vi "TSCAN_DBC_R&S.vi"(10 "Data":T4={"Communication message"={"Sender"="", "receiver"="", "message"="", "data"=variant}, "Data"={"Config_parameter"={"Bus_Type"=0, "Channel"=1, "Channels used"=1, "DLL_PATH"=path "", "Read message type"=1, "REC_Channel"=0}, "Send_parameter"={"SendData"=[0, 0, 0, 0, 0, 0, 0, 0, 0, 0, 0, 0, 0, 0, 0, 0, 0, 0, 0, 0, 0, 0, 0, 0, 0, 0, 0, 0, 0, 0, 0, 0, 0, 0, 0, 0, 0, 0, 0, 0, 0, 0, 0, 0, 0, 0, 0, 0, 0, 0, 0, 0, 0, 0, 0, 0, 0, 0, 0, 0, 0, 0, 0, 0, 0, 0, 0, 0, 0, 0, 0, 0, 0, 0, 0], "Data Length"=15, "ID"=0, "Frame Format"=0, "Frame Type"=0, "BRS"=enum."Close", "FD Frame"=0, "async&sync"=enum."async", "Timeout"=0}, "DBC_Ctr"={"DBC Path"=path "", "DBC loading channel"=0, "DatabaseId"=0, "DBMessages"=[], "DBSignals"=[]}, "CAN_Config_Array"=[], "CANFD_Config_Array"=[], "CAN_Config_Regs_Array"=[], "CANFD_Config_Regs_Array"=[], "Blf_Log"={"Blf_Log_PATH"=path ""}, "UDS"={"UDS Control"={"UDS Channel Index"=0, "Request ID"=1992, "Response ID"=2015, "Request ID (Func)"=1, "Session Mode"=1, "Reset Mode"=255, "DTC Mask"=0, "GropOfDTC"=0, "Seed Level"=2, "Seed"=[], "Key Level"=0, "Key"=[], "Read Identifier"=0, "UDS Read Data"=[], "ASCII Data"="", "Write Identifier"=0, "UDS Wrtie Data"=[], "IO Control Identifier"=1, "UDS IOControl Data"=[], "IO Control Mode"=0, "UDS IOControl Read Data"=[], "Routine Control Identifier"=0, "UDS RoutineControl Data"=[], "UDS RoutineControl Read Data"=[], "Routine Control Mode"=1, "SupportFDCAN"=TRUE, "time config"={"p2_timeout"=0, "p2_extended"=0, "s3_servertime"=0, "s3_clienttime"=0}, "ServiceLayer"={"FilledByte"=0, "STMin"=10, "BlockSize"=10, "FCDelay"=10, "MaxLength"=4095}, "Request"=[], "Respond"=[]}, "DiagModuleIndex"=1984}}, "CAN_Buffer"=[], "CANFD_Buffer"=[], "error in"={"status"=FALSE, "code"=0, "source"=""}, "CAN_Period_Datas"=[], "CANFD_period_Datas"=[], "CAN_Filtering_Datas"=[], "CANFD_Filtering_Datas"=[], "AsynCall?"=FALSE} {"Data"."UDS"."UDS Control"."Respond" format="%.0x"; "Data"."UDS"."UDS Control"."Request" format="%.0x"; "Data"."UDS"."UDS Control"."ServiceLayer"."FilledByte" format="%.0x"; "Data"."UDS"."UDS Control"."GropOfDTC" format="%.0x"; "Data"."UDS"."UDS Control"."DTC Mask" format="%.0x"; "Data"."UDS"."UDS Control"."UDS RoutineControl Read Data" format="%.0x"; "Data"."UDS"."UDS Control"."UDS RoutineControl Data" format="%.0x"; "Data"."UDS"."UDS Control"."Routine Control Identifier" format="%.0x"; "Data"."UDS"."UDS Control"."UDS IOControl Read Data" format="%.0x"; "Data"."UDS"."UDS Control"."UDS IOControl Data" format="%.0x"; "Data"."UDS"."UDS Control"."IO Control Identifier" format="%.0x"; "Data"."UDS"."UDS Control"."UDS Wrtie Data" format="%.0x"; "Data"."UDS"."UDS Control"."UDS Read Data" format="%.0x"; "Data"."UDS"."UDS Control"."Write Identifier" format="%.0x"; "Data"."UDS"."UDS Control"."Read Identifier" format="%.0x"; "Data"."UDS"."UDS Control"."Key" format="%.0x"; "Data"."UDS"."UDS Control"."Seed" format="%.0x"; "Data"."UDS"."UDS Control"."Request ID (Func)" format="%.0x"; "Data"."UDS"."UDS Control"."Response ID" format="%.0x"; "Data"."UDS"."UDS Control"."Request ID" format="%.0x"; "Data"."UDS"."UDS Control"."Session Mode" items=["DefaultSession"=1, "ProgrammingSession"=2, "ExtendedDiagnosticSession"=3]; "Data"."UDS"."UDS Control"."Reset Mode" items=["HardReset"=1, "keyOffOnReset"=2, "SoftReset"=3]; "Data"."UDS"."UDS Control"."IO Control Mode" items=["ReturnControlToECU", "ResetToDefault", "FreezeCurrentState", "ShortTermAdjustment"]; "Data"."UDS"."UDS Control"."Routine Control Mode" items=["Start routine"=1, "Stop routine"=2, "Request routine results"=3]; "Data"."CAN_Config_Regs_Array"."CAN configuration"."AAppChannel" items=["CHN1", "CHN2", "CHN3", "CHN4", "CHN5", "CHN6", "CHN7", "CHN8", "CHN9", "CHN10", "CHN11", "CHN12", "CHN13", "CHN14", "CHN15", "CHN16", "CHN17", "CHN18", "CHN19", "CHN20", "CHN21", "CHN22", "CHN23", "CHN24", "CHN25", "CHN26", "CHN27", "CHN28", "CHN29", "CHN30", "CHN31", "CHN32"]; "Data"."CAN_Config_Regs_Array"."CAN configuration"."AHwChannel" items=["CHN1", "CHN2", "CHN3", "CHN4", "CHN5", "CHN6", "CHN7", "CHN8", "CHN9", "CHN10", "CHN11", "CHN12", "CHN13", "CHN14", "CHN15", "CHN16", "CHN17", "CHN18", "CHN19", "CHN20", "CHN21", "CHN22", "CHN23", "CHN24", "CHN25", "CHN26", "CHN27", "CHN28", "CHN29", "CHN30", "CHN31", "CHN32"]; "Data"."CAN_Config_Regs_Array"."CAN configuration"."HardwareType" items=["BUS_UNKNOWN_TYPE", "TS_TCP_DEVICE", "XL_USB_DEVICE", "TS_USB_DEVICE", "PEAK_USB_DEVICE", "KVASER_USB_DEVICE", "ZLG_USB_DEVICE", "ICS_USB_DEVICE", "TS_TC1005_DEVICE", "CANABLE_USB_DEVICE", "TS_WIRELESS_OBD", "TS_USB_DEVICE_EX", "IXXAT_USB_DEVICE", "TS_ETH_IF_DEVICE", "TS_USB_IF_DEVICE", "BUS_DEV_TYPE_COUNT"]; "Data"."CANFD_Config_Regs_Array"."CANFD Configuration"."Hardware Type" items=["BUS_UNKNOWN_TYPE", "TS_TCP_DEVICE", "XL_USB_DEVICE", "TS_USB_DEVICE", "PEAK_USB_DEVICE", "KVASER_USB_DEVICE", "ZLG_USB_DEVICE", "ICS_USB_DEVICE", "TS_TC1005_DEVICE", "CANABLE_USB_DEVICE", "TS_WIRELESS_OBD", "TS_USB_DEVICE_EX", "IXXAT_USB_DEVICE", "TS_ETH_IF_DEVICE", "TS_USB_IF_DEVICE", "BUS_DEV_TYPE_COUNT"]; "Data"."CANFD_Config_Regs_Array"."CANFD Configuration"."AHwChannel" items=["CHN1", "CHN2", "CHN3", "CHN4", "CHN5", "CHN6", "CHN7", "CHN8", "CHN9", "CHN10", "CHN11", "CHN12", "CHN13", "CHN14", "CHN15", "CHN16", "CHN17", "CHN18", "CHN19", "CHN20", "CHN21", "CHN22", "CHN23", "CHN24", "CHN25", "CHN26", "CHN27", "CHN28", "CHN29", "CHN30", "CHN31", "CHN32"]; "Data"."CANFD_Config_Regs_Array"."CANFD Configuration"."AAppChannel" items=["CHN1", "CHN2", "CHN3", "CHN4", "CHN5", "CHN6", "CHN7", "CHN8", "CHN9", "CHN10", "CHN11", "CHN12", "CHN13", "CHN14", "CHN15", "CHN16", "CHN17", "CHN18", "CHN19", "CHN20", "CHN21", "CHN22", "CHN23", "CHN24", "CHN25", "CHN26", "CHN27", "CHN28", "CHN29", "CHN30", "CHN31", "CHN32"]; "Data"."CANFD_Config_Regs_Array"."CANFD Configuration"."AControllerType" items=["lfdtCAN", "lfdtISOFDCAN", "lfdtNonISOFDFDCAN"]; "Data"."CANFD_Config_Regs_Array"."CANFD Configuration"."AControllerMode" items=["lfdmNormal", "lfdmACKOff", "lfdmRestricted"]; "Data"."CANFD_Config_Array"."Hardware Type" items=["BUS_UNKNOWN_TYPE", "TS_TCP_DEVICE", "XL_USB_DEVICE", "TS_USB_DEVICE", "PEAK_USB_DEVICE", "KVASER_USB_DEVICE", "ZLG_USB_DEVICE", "ICS_USB_DEVICE", "TS_TC1005_DEVICE", "CANABLE_USB_DEVICE", "TS_WIRELESS_OBD", "TS_USB_DEVICE_EX", "IXXAT_USB_DEVICE", "TS_ETH_IF_DEVICE", "TS_USB_IF_DEVICE", "BUS_DEV_TYPE_COUNT"]; "Data"."CANFD_Config_Array"."AHwChannel" items=["CHN1", "CHN2", "CHN3", "CHN4", "CHN5", "CHN6", "CHN7", "CHN8", "CHN9", "CHN10", "CHN11", "CHN12", "CHN13", "CHN14", "CHN15", "CHN16", "CHN17", "CHN18", "CHN19", "CHN20", "CHN21", "CHN22", "CHN23", "CHN24", "CHN25", "CHN26", "CHN27", "CHN28", "CHN29", "CHN30", "CHN31", "CHN32"]; "Data"."CANFD_Config_Array"."AAppChannel" items=["CHN1", "CHN2", "CHN3", "CHN4", "CHN5", "CHN6", "CHN7", "CHN8", "CHN9", "CHN10", "CHN11", "CHN12", "CHN13", "CHN14", "CHN15", "CHN16", "CHN17", "CHN18", "CHN19", "CHN20", "CHN21", "CHN22", "CHN23", "CHN24", "CHN25", "CHN26", "CHN27", "CHN28", "CHN29", "CHN30", "CHN31", "CHN32"]; "Data"."CANFD_Config_Array"."AControllerType" items=["lfdtCAN", "lfdtISOFDCAN", "lfdtNonISOFDFDCAN"]; "Data"."CANFD_Config_Array"."AControllerMode" items=["lfdmNormal", "lfdmACKOff", "lfdmRestricted"]; "Data"."CAN_Config_Array"."AAppChannel" items=["CHN1", "CHN2", "CHN3", "CHN4", "CHN5", "CHN6", "CHN7", "CHN8", "CHN9", "CHN10", "CHN11", "CHN12", "CHN13", "CHN14", "CHN15", "CHN16", "CHN17", "CHN18", "CHN19", "CHN20", "CHN21", "CHN22", "CHN23", "CHN24", "CHN25", "CHN26", "CHN27", "CHN28", "CHN29", "CHN30", "CHN31", "CHN32"]; "Data"."CAN_Config_Array"."AHwChannel" items=["CHN1", "CHN2", "CHN3", "CHN4", "CHN5", "CHN6", "CHN7", "CHN8", "CHN9", "CHN10", "CHN11", "CHN12", "CHN13", "CHN14", "CHN15", "CHN16", "CHN17", "CHN18", "CHN19", "CHN20", "CHN21", "CHN22", "CHN23", "CHN24", "CHN25", "CHN26", "CHN27", "CHN28", "CHN29", "CHN30", "CHN31", "CHN32"]; "Data"."CAN_Config_Array"."HardwareType" items=["BUS_UNKNOWN_TYPE", "TS_TCP_DEVICE", "XL_USB_DEVICE", "TS_USB_DEVICE", "PEAK_USB_DEVICE", "KVASER_USB_DEVICE", "ZLG_USB_DEVICE", "ICS_USB_DEVICE", "TS_TC1005_DEVICE", "CANABLE_USB_DEVICE", "TS_WIRELESS_OBD", "TS_USB_DEVICE_EX", "IXXAT_USB_DEVICE", "TS_ETH_IF_DEVICE", "TS_USB_IF_DEVICE", "BUS_DEV_TYPE_COUNT"]; "Data"."DBC_Ctr"."DBSignals"."SignalList"."Message_Type" items=["CAN", "CANFD", "J1939"]; "Data"."DBC_Ctr"."DBSignals"."SignalList"."Mux_Type" items=["Normal", "multiplexor", "multiplexed"]; "Data"."DBC_Ctr"."DBSignals"."SignalList"."Is_Motorola" items=["Intel", "Motorola"]; "Data"."DBC_Ctr"."DBSignals"."SignalList"."Value_Type" items=["unsigned int", "signed int", "float", "double"]; "Data"."DBC_Ctr"."DBSignals"."SignalList"."ID" format="%.0x"; "Data"."DBC_Ctr"."DBMessages"."BRS" items=["No BRS", "BRS"]; "Data"."DBC_Ctr"."DBMessages"."ID" format="%.0x"; "Data"."DBC_Ctr"."DBMessages"."Type" items=["cftStdCAN", "cftExtCAN", "cftJ1939", "cftStdCANFD", "cftExtCANFD"]; "Data"."DBC_Ctr"."DBC loading channel" items=["CHN1", "CHN2", "CHN3", "CHN4", "CHN5", "CHN6", "CHN7", "CHN8", "CHN9", "CHN10", "CHN11", "CHN12", "CHN13", "CHN14", "CHN15", "CHN16", "CHN17", "CHN18", "CHN19", "CHN20", "CHN21", "CHN22", "CHN23", "CHN24", "CHN25", "CHN26", "CHN27", "CHN28", "CHN29", "CHN30", "CHN31", "CHN32"]; "Data"."Send_parameter"."FD Frame" items=["Ordinary CAN Data", "FD CAN Data"]; "Data"."Send_parameter"."Frame Type" items=["Standard Frame", "Extended Frame"]; "Data"."Send_parameter"."Frame Format" items=["Standard Frame", "Extended Frame"]; "Data"."Send_parameter"."ID" format="%x"; "Data"."Send_parameter"."Data Length" items=["0", "1", "2", "3", "4", "5", "6", "7", "8", "12", "16", "20", "24", "32", "48", "64"]; "Data"."Send_parameter"."SendData" format="%x"; "Data"."Config_parameter"."REC_Channel" items=["CHN1", "CHN2", "CHN3", "CHN4", "CHN5", "CHN6", "CHN7", "CHN8", "CHN9", "CHN10", "CHN11", "CHN12", "CHN13", "CHN14", "CHN15", "CHN16", "CHN17", "CHN18", "CHN19", "CHN20", "CHN21", "CHN22", "CHN23", "CHN24", "CHN25", "CHN26", "CHN27", "CHN28", "CHN29", "CHN30", "CHN31", "CHN32"]; "Data"."Config_parameter"."Read message type" items=["Only read received messages", "Receive&send messages"]; "Data"."Config_parameter"."Channels used" items=["1 Channel"=1, "2 Channels"=2, "3 Channels"=3, "4 Channels"=4, "5 Channels"=5, "6 Channels"=6, "7 Channels"=7, "8 Channels"=8, "9 Channels"=9, "10 Channels"=10, "11 Channels"=11, "12 Channels"=12, "13 Channels"=13, "14 Channels"=14, "15 Channels"=15, "16 Channels"=16]; "Data"."Config_parameter"."Channel" items=["Disable", "Enable"]; "Data"."Config_parameter"."Bus_Type" items=["CAN", "CANFD"]}, 11 "Sender":string="Demo") -> (2 "Data 2":T4={"Communication message"={"Sender"="", "receiver"="", "message"="", "data"=variant}, "Data"={"Config_parameter"={"Bus_Type"=0, "Channel"=1, "Channels used"=1, "DLL_PATH"=path "", "Read message type"=1, "REC_Channel"=0}, "Send_parameter"={"SendData"=[0, 0, 0, 0, 0, 0, 0, 0, 0, 0, 0, 0, 0, 0, 0, 0, 0, 0, 0, 0, 0, 0, 0, 0, 0, 0, 0, 0, 0, 0, 0, 0, 0, 0, 0, 0, 0, 0, 0, 0, 0, 0, 0, 0, 0, 0, 0, 0, 0, 0, 0, 0, 0, 0, 0, 0, 0, 0, 0, 0, 0, 0, 0, 0, 0, 0, 0, 0, 0, 0, 0, 0, 0, 0, 0], "Data Length"=15, "ID"=0, "Frame Format"=0, "Frame Type"=0, "BRS"=enum."Close", "FD Frame"=0, "async&sync"=enum."async", "Timeout"=0}, "DBC_Ctr"={"DBC Path"=path "", "DBC loading channel"=0, "DatabaseId"=0, "DBMessages"=[], "DBSignals"=[]}, "CAN_Config_Array"=[], "CANFD_Config_Array"=[], "CAN_Config_Regs_Array"=[], "CANFD_Config_Regs_Array"=[], "Blf_Log"={"Blf_Log_PATH"=path ""}, "UDS"={"UDS Control"={"UDS Channel Index"=0, "Request ID"=1992, "Response ID"=2015, "Request ID (Func)"=1, "Session Mode"=1, "Reset Mode"=255, "DTC Mask"=0, "GropOfDTC"=0, "Seed Level"=2, "Seed"=[], "Key Level"=0, "Key"=[], "Read Identifier"=0, "UDS Read Data"=[], "ASCII Data"="", "Write Identifier"=0, "UDS Wrtie Data"=[], "IO Control Identifier"=1, "UDS IOControl Data"=[], "IO Control Mode"=0, "UDS IOControl Read Data"=[], "Routine Control Identifier"=0, "UDS RoutineControl Data"=[], "UDS RoutineControl Read Data"=[], "Routine Control Mode"=1, "SupportFDCAN"=TRUE, "time config"={"p2_timeout"=0, "p2_extended"=0, "s3_servertime"=0, "s3_clienttime"=0}, "ServiceLayer"={"FilledByte"=0, "STMin"=10, "BlockSize"=10, "FCDelay"=10, "MaxLength"=4095}, "Request"=[], "Respond"=[]}, "DiagModuleIndex"=1984}}, "CAN_Buffer"=[], "CANFD_Buffer"=[], "error in"={"status"=FALSE, "code"=0, "source"=""}, "CAN_Period_Datas"=[], "CANFD_period_Datas"=[], "CAN_Filtering_Datas"=[], "CANFD_Filtering_Datas"=[], "AsynCall?"=FALSE} {"Data"."UDS"."UDS Control"."Respond" format="%.0x"; "Data"."UDS"."UDS Control"."Request" format="%.0x"; "Data"."UDS"."UDS Control"."ServiceLayer"."FilledByte" format="%.0x"; "Data"."UDS"."UDS Control"."GropOfDTC" format="%.0x"; "Data"."UDS"."UDS Control"."DTC Mask" format="%.0x"; "Data"."UDS"."UDS Control"."UDS RoutineControl Read Data" format="%.0x"; "Data"."UDS"."UDS Control"."UDS RoutineControl Data" format="%.0x"; "Data"."UDS"."UDS Control"."Routine Control Identifier" format="%.0x"; "Data"."UDS"."UDS Control"."UDS IOControl Read Data" format="%.0x"; "Data"."UDS"."UDS Control"."UDS IOControl Data" format="%.0x"; "Data"."UDS"."UDS Control"."IO Control Identifier" format="%.0x"; "Data"."UDS"."UDS Control"."UDS Wrtie Data" format="%.0x"; "Data"."UDS"."UDS Control"."UDS Read Data" format="%.0x"; "Data"."UDS"."UDS Control"."Write Identifier" format="%.0x"; "Data"."UDS"."UDS Control"."Read Identifier" format="%.0x"; "Data"."UDS"."UDS Control"."Key" format="%.0x"; "Data"."UDS"."UDS Control"."Seed" format="%.0x"; "Data"."UDS"."UDS Control"."Request ID (Func)" format="%.0x"; "Data"."UDS"."UDS Control"."Response ID" format="%.0x"; "Data"."UDS"."UDS Control"."Request ID" format="%.0x"; "Data"."UDS"."UDS Control"."Session Mode" items=["DefaultSession"=1, "ProgrammingSession"=2, "ExtendedDiagnosticSession"=3]; "Data"."UDS"."UDS Control"."Reset Mode" items=["HardReset"=1, "keyOffOnReset"=2, "SoftReset"=3]; "Data"."UDS"."UDS Control"."IO Control Mode" items=["ReturnControlToECU", "ResetToDefault", "FreezeCurrentState", "ShortTermAdjustment"]; "Data"."UDS"."UDS Control"."Routine Control Mode" items=["Start routine"=1, "Stop routine"=2, "Request routine results"=3]; "Data"."CAN_Config_Regs_Array"."CAN configuration"."AAppChannel" items=["CHN1", "CHN2", "CHN3", "CHN4", "CHN5", "CHN6", "CHN7", "CHN8", "CHN9", "CHN10", "CHN11", "CHN12", "CHN13", "CHN14", "CHN15", "CHN16", "CHN17", "CHN18", "CHN19", "CHN20", "CHN21", "CHN22", "CHN23", "CHN24", "CHN25", "CHN26", "CHN27", "CHN28", "CHN29", "CHN30", "CHN31", "CHN32"]; "Data"."CAN_Config_Regs_Array"."CAN configuration"."AHwChannel" items=["CHN1", "CHN2", "CHN3", "CHN4", "CHN5", "CHN6", "CHN7", "CHN8", "CHN9", "CHN10", "CHN11", "CHN12", "CHN13", "CHN14", "CHN15", "CHN16", "CHN17", "CHN18", "CHN19", "CHN20", "CHN21", "CHN22", "CHN23", "CHN24", "CHN25", "CHN26", "CHN27", "CHN28", "CHN29", "CHN30", "CHN31", "CHN32"]; "Data"."CAN_Config_Regs_Array"."CAN configuration"."HardwareType" items=["BUS_UNKNOWN_TYPE", "TS_TCP_DEVICE", "XL_USB_DEVICE", "TS_USB_DEVICE", "PEAK_USB_DEVICE", "KVASER_USB_DEVICE", "ZLG_USB_DEVICE", "ICS_USB_DEVICE", "TS_TC1005_DEVICE", "CANABLE_USB_DEVICE", "TS_WIRELESS_OBD", "TS_USB_DEVICE_EX", "IXXAT_USB_DEVICE", "TS_ETH_IF_DEVICE", "TS_USB_IF_DEVICE", "BUS_DEV_TYPE_COUNT"]; "Data"."CANFD_Config_Regs_Array"."CANFD Configuration"."Hardware Type" items=["BUS_UNKNOWN_TYPE", "TS_TCP_DEVICE", "XL_USB_DEVICE", "TS_USB_DEVICE", "PEAK_USB_DEVICE", "KVASER_USB_DEVICE", "ZLG_USB_DEVICE", "ICS_USB_DEVICE", "TS_TC1005_DEVICE", "CANABLE_USB_DEVICE", "TS_WIRELESS_OBD", "TS_USB_DEVICE_EX", "IXXAT_USB_DEVICE", "TS_ETH_IF_DEVICE", "TS_USB_IF_DEVICE", "BUS_DEV_TYPE_COUNT"]; "Data"."CANFD_Config_Regs_Array"."CANFD Configuration"."AHwChannel" items=["CHN1", "CHN2", "CHN3", "CHN4", "CHN5", "CHN6", "CHN7", "CHN8", "CHN9", "CHN10", "CHN11", "CHN12", "CHN13", "CHN14", "CHN15", "CHN16", "CHN17", "CHN18", "CHN19", "CHN20", "CHN21", "CHN22", "CHN23", "CHN24", "CHN25", "CHN26", "CHN27", "CHN28", "CHN29", "CHN30", "CHN31", "CHN32"]; "Data"."CANFD_Config_Regs_Array"."CANFD Configuration"."AAppChannel" items=["CHN1", "CHN2", "CHN3", "CHN4", "CHN5", "CHN6", "CHN7", "CHN8", "CHN9", "CHN10", "CHN11", "CHN12", "CHN13", "CHN14", "CHN15", "CHN16", "CHN17", "CHN18", "CHN19", "CHN20", "CHN21", "CHN22", "CHN23", "CHN24", "CHN25", "CHN26", "CHN27", "CHN28", "CHN29", "CHN30", "CHN31", "CHN32"]; "Data"."CANFD_Config_Regs_Array"."CANFD Configuration"."AControllerType" items=["lfdtCAN", "lfdtISOFDCAN", "lfdtNonISOFDFDCAN"]; "Data"."CANFD_Config_Regs_Array"."CANFD Configuration"."AControllerMode" items=["lfdmNormal", "lfdmACKOff", "lfdmRestricted"]; "Data"."CANFD_Config_Array"."Hardware Type" items=["BUS_UNKNOWN_TYPE", "TS_TCP_DEVICE", "XL_USB_DEVICE", "TS_USB_DEVICE", "PEAK_USB_DEVICE", "KVASER_USB_DEVICE", "ZLG_USB_DEVICE", "ICS_USB_DEVICE", "TS_TC1005_DEVICE", "CANABLE_USB_DEVICE", "TS_WIRELESS_OBD", "TS_USB_DEVICE_EX", "IXXAT_USB_DEVICE", "TS_ETH_IF_DEVICE", "TS_USB_IF_DEVICE", "BUS_DEV_TYPE_COUNT"]; "Data"."CANFD_Config_Array"."AHwChannel" items=["CHN1", "CHN2", "CHN3", "CHN4", "CHN5", "CHN6", "CHN7", "CHN8", "CHN9", "CHN10", "CHN11", "CHN12", "CHN13", "CHN14", "CHN15", "CHN16", "CHN17", "CHN18", "CHN19", "CHN20", "CHN21", "CHN22", "CHN23", "CHN24", "CHN25", "CHN26", "CHN27", "CHN28", "CHN29", "CHN30", "CHN31", "CHN32"]; "Data"."CANFD_Config_Array"."AAppChannel" items=["CHN1", "CHN2", "CHN3", "CHN4", "CHN5", "CHN6", "CHN7", "CHN8", "CHN9", "CHN10", "CHN11", "CHN12", "CHN13", "CHN14", "CHN15", "CHN16", "CHN17", "CHN18", "CHN19", "CHN20", "CHN21", "CHN22", "CHN23", "CHN24", "CHN25", "CHN26", "CHN27", "CHN28", "CHN29", "CHN30", "CHN31", "CHN32"]; "Data"."CANFD_Config_Array"."AControllerType" items=["lfdtCAN", "lfdtISOFDCAN", "lfdtNonISOFDFDCAN"]; "Data"."CANFD_Config_Array"."AControllerMode" items=["lfdmNormal", "lfdmACKOff", "lfdmRestricted"]; "Data"."CAN_Config_Array"."AAppChannel" items=["CHN1", "CHN2", "CHN3", "CHN4", "CHN5", "CHN6", "CHN7", "CHN8", "CHN9", "CHN10", "CHN11", "CHN12", "CHN13", "CHN14", "CHN15", "CHN16", "CHN17", "CHN18", "CHN19", "CHN20", "CHN21", "CHN22", "CHN23", "CHN24", "CHN25", "CHN26", "CHN27", "CHN28", "CHN29", "CHN30", "CHN31", "CHN32"]; "Data"."CAN_Config_Array"."AHwChannel" items=["CHN1", "CHN2", "CHN3", "CHN4", "CHN5", "CHN6", "CHN7", "CHN8", "CHN9", "CHN10", "CHN11", "CHN12", "CHN13", "CHN14", "CHN15", "CHN16", "CHN17", "CHN18", "CHN19", "CHN20", "CHN21", "CHN22", "CHN23", "CHN24", "CHN25", "CHN26", "CHN27", "CHN28", "CHN29", "CHN30", "CHN31", "CHN32"]; "Data"."CAN_Config_Array"."HardwareType" items=["BUS_UNKNOWN_TYPE", "TS_TCP_DEVICE", "XL_USB_DEVICE", "TS_USB_DEVICE", "PEAK_USB_DEVICE", "KVASER_USB_DEVICE", "ZLG_USB_DEVICE", "ICS_USB_DEVICE", "TS_TC1005_DEVICE", "CANABLE_USB_DEVICE", "TS_WIRELESS_OBD", "TS_USB_DEVICE_EX", "IXXAT_USB_DEVICE", "TS_ETH_IF_DEVICE", "TS_USB_IF_DEVICE", "BUS_DEV_TYPE_COUNT"]; "Data"."DBC_Ctr"."DBSignals"."SignalList"."Message_Type" items=["CAN", "CANFD", "J1939"]; "Data"."DBC_Ctr"."DBSignals"."SignalList"."Mux_Type" items=["Normal", "multiplexor", "multiplexed"]; "Data"."DBC_Ctr"."DBSignals"."SignalList"."Is_Motorola" items=["Intel", "Motorola"]; "Data"."DBC_Ctr"."DBSignals"."SignalList"."Value_Type" items=["unsigned int", "signed int", "float", "double"]; "Data"."DBC_Ctr"."DBSignals"."SignalList"."ID" format="%.0x"; "Data"."DBC_Ctr"."DBMessages"."BRS" items=["No BRS", "BRS"]; "Data"."DBC_Ctr"."DBMessages"."ID" format="%.0x"; "Data"."DBC_Ctr"."DBMessages"."Type" items=["cftStdCAN", "cftExtCAN", "cftJ1939", "cftStdCANFD", "cftExtCANFD"]; "Data"."DBC_Ctr"."DBC loading channel" items=["CHN1", "CHN2", "CHN3", "CHN4", "CHN5", "CHN6", "CHN7", "CHN8", "CHN9", "CHN10", "CHN11", "CHN12", "CHN13", "CHN14", "CHN15", "CHN16", "CHN17", "CHN18", "CHN19", "CHN20", "CHN21", "CHN22", "CHN23", "CHN24", "CHN25", "CHN26", "CHN27", "CHN28", "CHN29", "CHN30", "CHN31", "CHN32"]; "Data"."Send_parameter"."FD Frame" items=["Ordinary CAN Data", "FD CAN Data"]; "Data"."Send_parameter"."Frame Type" items=["Standard Frame", "Extended Frame"]; "Data"."Send_parameter"."Frame Format" items=["Standard Frame", "Extended Frame"]; "Data"."Send_parameter"."ID" format="%x"; "Data"."Send_parameter"."Data Length" items=["0", "1", "2", "3", "4", "5", "6", "7", "8", "12", "16", "20", "24", "32", "48", "64"]; "Data"."Send_parameter"."SendData" format="%x"; "Data"."Config_parameter"."REC_Channel" items=["CHN1", "CHN2", "CHN3", "CHN4", "CHN5", "CHN6", "CHN7", "CHN8", "CHN9", "CHN10", "CHN11", "CHN12", "CHN13", "CHN14", "CHN15", "CHN16", "CHN17", "CHN18", "CHN19", "CHN20", "CHN21", "CHN22", "CHN23", "CHN24", "CHN25", "CHN26", "CHN27", "CHN28", "CHN29", "CHN30", "CHN31", "CHN32"]; "Data"."Config_parameter"."Read message type" items=["Only read received messages", "Receive&send messages"]; "Data"."Config_parameter"."Channels used" items=["1 Channel"=1, "2 Channels"=2, "3 Channels"=3, "4 Channels"=4, "5 Channels"=5, "6 Channels"=6, "7 Channels"=7, "8 Channels"=8, "9 Channels"=9, "10 Channels"=10, "11 Channels"=11, "12 Channels"=12, "13 Channels"=13, "14 Channels"=14, "15 Channels"=15, "16 Channels"=16]; "Data"."Config_parameter"."Channel" items=["Disable", "Enable"]; "Data"."Config_parameter"."Bus_Type" items=["CAN", "CANFD"]})   [LabVIEW 2014]
uses:
  <vilib>/Utility/miscctls.llb/LVPointTypeDef.ctl
  Typedef/TLibCANFD.ctl
  Typedef/TLibCAN.ctl
  Typedef/TSCAN_Config_parameter.ctl
  Typedef/TSCAN_Send_parameter.ctl
  DataBase/Typedef/DBMessage.ctl
  DataBase/Typedef/DBSignal.ctl
  Typedef/TSCAN_DBC_Ctr.ctl
  All_Control/Typedef/Hardware Type.ctl
  Utilities/Typedef/Hardware_Subtype.ctl
  Typedef/TSCAN_CAN_Configuration.ctl
  Typedef/TSCAN_CANFD_Configuration.ctl
  Typedef/TSCAN_CANFD_Configuration_Regs.ctl
  Typedef/TSCAN_CAN_Configuration_Regs.ctl
  All_Control/Typedef/Blf_Log.ctl
  Diagnosis/Typedef/UDS Control.ctl
  Diagnosis/Typedef/UDS Cluster.ctl
  Typedef/TSCAN_CAN_CANFD_Demo_Data.ctl
  Typedef/TSCAN_CAN_CANFD_Demo_Data1.ctl
panel:
  out "Type":T1(ring)
  in  "Channel":i32(ring) items=["CHN1", "CHN2", "CHN3", "CHN4", "CHN5", "CHN6", "CHN7", "CHN8", "CHN9", "CHN10", "CHN11", "CHN12", "CHN13", "CHN14", "CHN15", "CHN16", "CHN17", "CHN18", "CHN19", "CHN20", "CHN21", "CHN22", "CHN23", "CHN24", "CHN25", "CHN26", "CHN27", "CHN28", "CHN29", "CHN30", "CHN31", "CHN32"]
  in  "Send":bool
  out "CANFD Data":T2 {"FIdentifier" format="%x"}
  out "CAN Data":T3 {"FIdentifier" format="%x"}
  in  "Signals":string[][](array[string])
  in  "Messages":string(combo)
  in  "Creat error":bool
  in  "log":i32(listbox)
  in  "Quit":bool
  # "Name"
  # "Value"
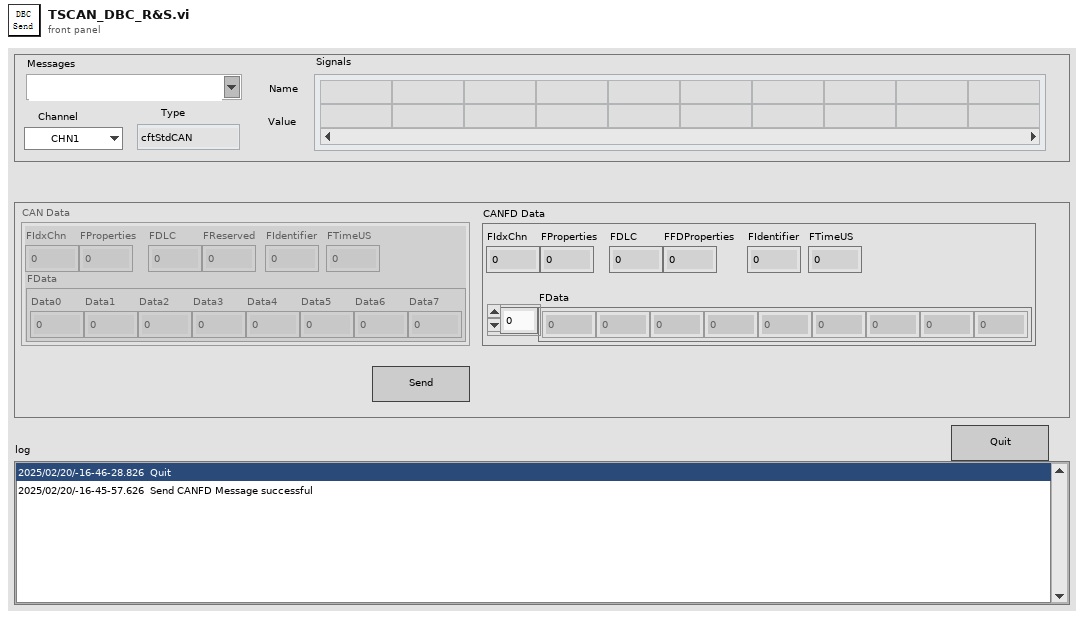
[diagram p1: front panel]
types:
  T1 = enum16{"cftStdCAN", "cftExtCAN", "cftJ1939", "cftStdCANFD", "cftExtCANFD"}
  T2 = cluster{"FIdxChn":u8, "FProperties":u8, "FDLC":u8, "FFDProperties":u8, "FIdentifier":i32, "FTimeUS":u64, "FData":dbl[]}
  T3 = cluster{"FIdxChn":u8, "FProperties":u8, "FDLC":u8, "FReserved":u8, "FIdentifier":i32, "FTimeUS":u64, "FData":cluster{"Data0":u8, "Data1":u8, "Data2":u8, "Data3":u8, "Data4":u8, "Data5":u8, "Data6":u8, "Data7":u8}}
  T4 = typedef "TSCAN_CAN_CANFD_Demo_Data1.ctl" = cluster{"Communication message":cluster{"Sender":string, "receiver":string, "message":string, "data":variant}, "Data":T5, "CAN_Buffer":cluster{"FIdxChn":u8, "FProperties":u8, "FDLC":u8, "FReserved":u8, "FIdentifier":i32, "FTimeUS":u64, "FData":cluster{"Data0":u8, "Data1":u8, "Data2":u8, "Data3":u8, "Data4":u8, "Data5":u8, "Data6":u8, "Data7":u8}}[], "CANFD_Buffer":cluster{"FIdxChn":u8, "FProperties":u8, "FDLC":u8, "FReserved":u8, "FIdentifier":i32, "FTimeUS":u64, "FDatas":cluster{"Initialize array[0]":u8, "Initialize array[1]":u8, "Initialize array[2]":u8, "Initialize array[3]":u8, "Initialize array[4]":u8, "Initialize array[5]":u8, "Initialize array[6]":u8, "Initialize array[7]":u8, "Initialize array[8]":u8, "Initialize array[9]":u8, "Initialize array[10]":u8, "Initialize array[11]":u8, "Initialize array[12]":u8, "Initialize array[13]":u8, "Initialize array[14]":u8, "Initialize array[15]":u8, "Initialize array[16]":u8, "Initialize array[17]":u8, "Initialize array[18]":u8, "Initialize array[19]":u8, "Initialize array[20]":u8, "Initialize array[21]":u8, "Initialize array[22]":u8, "Initialize array[23]":u8, "Initialize array[24]":u8, "Initialize array[25]":u8, "Initialize array[26]":u8, "Initialize array[27]":u8, "Initialize array[28]":u8, "Initialize array[29]":u8, "Initialize array[30]":u8, "Initialize array[31]":u8, "Initialize array[32]":u8, "Initialize array[33]":u8, "Initialize array[34]":u8, "Initialize array[35]":u8, "Initialize array[36]":u8, "Initialize array[37]":u8, "Initialize array[38]":u8, "Initialize array[39]":u8, "Initialize array[40]":u8, "Initialize array[41]":u8, "Initialize array[42]":u8, "Initialize array[43]":u8, "Initialize array[44]":u8, "Initialize array[45]":u8, "Initialize array[46]":u8, "Initialize array[47]":u8, "Initialize array[48]":u8, "Initialize array[49]":u8, "Initialize array[50]":u8, "Initialize array[51]":u8, "Initialize array[52]":u8, "Initialize array[53]":u8, "Initialize array[54]":u8, "Initialize array[55]":u8, "Initialize array[56]":u8, "Initialize array[57]":u8, "Initialize array[58]":u8, "Initialize array[59]":u8, "Initialize array[60]":u8, "Initialize array[61]":u8, "Initialize array[62]":u8, "Initialize array[63]":u8}}[], "error in":errorcluster, "CAN_Period_Datas":cluster{"FIdxChn":u8, "FProperties":u8, "FDLC":u8, "FReserved":u8, "FIdentifier":i32, "FTimeUS":u64, "FData":cluster{"Data0":u8, "Data1":u8, "Data2":u8, "Data3":u8, "Data4":u8, "Data5":u8, "Data6":u8, "Data7":u8}}[], "CANFD_period_Datas":cluster{"FIdxChn":u8, "FProperties":u8, "FDLC":u8, "FReserved":u8, "FIdentifier":i32, "FTimeUS":u64, "FDatas":cluster{"Initialize array[0]":u8, "Initialize array[1]":u8, "Initialize array[2]":u8, "Initialize array[3]":u8, "Initialize array[4]":u8, "Initialize array[5]":u8, "Initialize array[6]":u8, "Initialize array[7]":u8, "Initialize array[8]":u8, "Initialize array[9]":u8, "Initialize array[10]":u8, "Initialize array[11]":u8, "Initialize array[12]":u8, "Initialize array[13]":u8, "Initialize array[14]":u8, "Initialize array[15]":u8, "Initialize array[16]":u8, "Initialize array[17]":u8, "Initialize array[18]":u8, "Initialize array[19]":u8, "Initialize array[20]":u8, "Initialize array[21]":u8, "Initialize array[22]":u8, "Initialize array[23]":u8, "Initialize array[24]":u8, "Initialize array[25]":u8, "Initialize array[26]":u8, "Initialize array[27]":u8, "Initialize array[28]":u8, "Initialize array[29]":u8, "Initialize array[30]":u8, "Initialize array[31]":u8, "Initialize array[32]":u8, "Initialize array[33]":u8, "Initialize array[34]":u8, "Initialize array[35]":u8, "Initialize array[36]":u8, "Initialize array[37]":u8, "Initialize array[38]":u8, "Initialize array[39]":u8, "Initialize array[40]":u8, "Initialize array[41]":u8, "Initialize array[42]":u8, "Initialize array[43]":u8, "Initialize array[44]":u8, "Initialize array[45]":u8, "Initialize array[46]":u8, "Initialize array[47]":u8, "Initialize array[48]":u8, "Initialize array[49]":u8, "Initialize array[50]":u8, "Initialize array[51]":u8, "Initialize array[52]":u8, "Initialize array[53]":u8, "Initialize array[54]":u8, "Initialize array[55]":u8, "Initialize array[56]":u8, "Initialize array[57]":u8, "Initialize array[58]":u8, "Initialize array[59]":u8, "Initialize array[60]":u8, "Initialize array[61]":u8, "Initialize array[62]":u8, "Initialize array[63]":u8}}[], "CAN_Filtering_Datas":cluster{"FIdxChn":u8, "FProperties":u8, "FDLC":u8, "FReserved":u8, "FIdentifier":i32, "FTimeUS":u64, "FData":cluster{"Data0":u8, "Data1":u8, "Data2":u8, "Data3":u8, "Data4":u8, "Data5":u8, "Data6":u8, "Data7":u8}}[], "CANFD_Filtering_Datas":cluster{"FIdxChn":u8, "FProperties":u8, "FDLC":u8, "FReserved":u8, "FIdentifier":i32, "FTimeUS":u64, "FDatas":cluster{"Initialize array[0]":u8, "Initialize array[1]":u8, "Initialize array[2]":u8, "Initialize array[3]":u8, "Initialize array[4]":u8, "Initialize array[5]":u8, "Initialize array[6]":u8, "Initialize array[7]":u8, "Initialize array[8]":u8, "Initialize array[9]":u8, "Initialize array[10]":u8, "Initialize array[11]":u8, "Initialize array[12]":u8, "Initialize array[13]":u8, "Initialize array[14]":u8, "Initialize array[15]":u8, "Initialize array[16]":u8, "Initialize array[17]":u8, "Initialize array[18]":u8, "Initialize array[19]":u8, "Initialize array[20]":u8, "Initialize array[21]":u8, "Initialize array[22]":u8, "Initialize array[23]":u8, "Initialize array[24]":u8, "Initialize array[25]":u8, "Initialize array[26]":u8, "Initialize array[27]":u8, "Initialize array[28]":u8, "Initialize array[29]":u8, "Initialize array[30]":u8, "Initialize array[31]":u8, "Initialize array[32]":u8, "Initialize array[33]":u8, "Initialize array[34]":u8, "Initialize array[35]":u8, "Initialize array[36]":u8, "Initialize array[37]":u8, "Initialize array[38]":u8, "Initialize array[39]":u8, "Initialize array[40]":u8, "Initialize array[41]":u8, "Initialize array[42]":u8, "Initialize array[43]":u8, "Initialize array[44]":u8, "Initialize array[45]":u8, "Initialize array[46]":u8, "Initialize array[47]":u8, "Initialize array[48]":u8, "Initialize array[49]":u8, "Initialize array[50]":u8, "Initialize array[51]":u8, "Initialize array[52]":u8, "Initialize array[53]":u8, "Initialize array[54]":u8, "Initialize array[55]":u8, "Initialize array[56]":u8, "Initialize array[57]":u8, "Initialize array[58]":u8, "Initialize array[59]":u8, "Initialize array[60]":u8, "Initialize array[61]":u8, "Initialize array[62]":u8, "Initialize array[63]":u8}}[], "AsynCall?":bool}
  T5 = typedef "TSCAN_CAN_CANFD_Demo_Data.ctl" = cluster{"Config_parameter":T6, "Send_parameter":T7, "DBC_Ctr":T8, "CAN_Config_Array":T11[], "CANFD_Config_Array":T14[], "CAN_Config_Regs_Array":T15[], "CANFD_Config_Regs_Array":T16[], "Blf_Log":T17, "UDS":T18}
  T6 = typedef "TSCAN_Config_parameter.ctl" = cluster{"Bus_Type":u16, "Channel":i32, "Channels used":u16, "DLL_PATH":path, "Read message type":u16, "REC_Channel":i32}
  T7 = typedef "TSCAN_Send_parameter.ctl" = cluster{"SendData":u8[], "Data Length":i32, "ID":i32, "Frame Format":u8, "Frame Type":u8, "BRS":enum16{"Close", "Open"}, "FD Frame":u8, "async&sync":enum16{"async", "sync"}, "Timeout":u16}
  T8 = typedef "TSCAN_DBC_Ctr.ctl" = cluster{"DBC Path":path, "DBC loading channel":i32, "DatabaseId":u32, "DBMessages":T9[], "DBSignals":cluster{"MessageName":string, "SignalList":T10[]}[]}
  T9 = typedef "DBMessage.ctl" = cluster{"Type":u16, "DLC":i32, "ID":i32, "CycleTime":dbl, "Name":string, "Comment":string, "TX_Node_Index":i32, "Owned_Signal_List_Count ":i32, "Owned_Signal_List_Signal_Index":i32, "BRS":i32}
  T10 = typedef "DBSignal.ctl" = cluster{"ID":i32, "Value_Type":i32, "Is_Motorola":i32, "ValTab_Index":i32, "Mux_Type":i32, "Mux_Value":dbl, "Layout_Start":i32, "Length":i32, "Factor":dbl, "Offset":dbl, "InitValue":dbl, "Min":dbl, "Max":dbl, "Name":string, "Unit":string, "Comment":string, "Message_Index":i32, "Message_Type":i32}
  T11 = typedef "TSCAN_CAN_Configuration.ctl" = cluster{"HardwareType":T12, "Hardware Subtype":T13, "ABaudrateKbps":sgl, "AListenOnly":enum16{"Normal", "ListenOnly"}, "Int120Ohm":enum16{"Disable", "Enable"}, "EnableChannel":enum16{"Disable", "Enable"}, "AHwChannel":i32, "AAppChannel":i32, "AldHW":i32}
  T12 = typedef "Hardware Type.ctl" = i32
  T13 = typedef "Hardware_Subtype.ctl" = enum16{"TS_UNKNOWN_DEVICE", "TSCAN_PRO", "TSCAN_Lite1", "TC1001", "TL1001", "TC1011", "TM5011", "TC1002", "TC1014", "TSCANFD2517", "TC1026", "TC1016", "TC1012", "TC1013", "TLog1002", "TC1034", "TC1018", "GW2116", "TC2115", "MP1013", "TC1113", "TC1114", "TP1013", "TC1017", "TP1018", "TF10XX", "TL1004_FD_4_LIN_2", "TE1051", "TP1051", "TP1034", "TTS9015", "TP1026", "TTS1026", "TTS1034", "TTS1018", "TL1011", "TTS1015_LiAuto", "TTS1013_LiAuto", "TTS1016Pro", "TC1054Pro", "TC1054", "TLog1038", "TO1013", "TC1034Pro", "TC1018Pro", "TC1038Pro", "TS_DEV_END"}
  T14 = typedef "TSCAN_CANFD_Configuration.ctl" = cluster{"Hardware Type":T12, "Hardware Subtype":T13, "AArbRateKbps":sgl, "AListenOnly":enum16{"Normal", "ListenOnly"}, "Int120Ohm":enum16{"Disable", "Enable"}, "EnableChannel":enum16{"Disable", "Enable"}, "AHwChannel":i32, "AAppChannel":i32, "ADataRateKbps":sgl, "AControllerType":i32, "AControllerMode":i32, "AldHW":i32}
  T15 = typedef "TSCAN_CAN_Configuration_Regs.ctl" = cluster{"CAN_Sampling point":cluster{"ASEG1":i32, "ASEG2":i32, "APrescaler":i32, "ASJW":i32}, "CAN configuration":T11}
  T16 = typedef "TSCAN_CANFD_Configuration_Regs.ctl" = cluster{"CANFD Configuration":T14, "CANFD_Sampling point":cluster{"AArbSEG1":i32, "AArbSEG2":i32, "AArbPrescaler":i32, "AArbSJW":i32, "ADataSEG1":i32, "ADataSEG2":i32, "ADataPrescaler":i32, "ADataSJW":i32}}
  T17 = typedef "Blf_Log.ctl" = cluster{"Blf_Log_PATH":path}
  T18 = typedef "UDS Cluster.ctl" = cluster{"UDS Control":T19, "DiagModuleIndex":i32}
  T19 = typedef "UDS Control.ctl" = cluster{"UDS Channel Index":u32, "Request ID":u32, "Response ID":u32, "Request ID (Func)":u32, "Session Mode":u8, "Reset Mode":u8, "DTC Mask":u8, "GropOfDTC":u32, "Seed Level":i32, "Seed":u8[], "Key Level":i32, "Key":u8[], "Read Identifier":u16, "UDS Read Data":u8[], "ASCII Data":string, "Write Identifier":u16, "UDS Wrtie Data":u8[], "IO Control Identifier":u16, "UDS IOControl Data":u8[], "IO Control Mode":u8, "UDS IOControl Read Data":u8[], "Routine Control Identifier":u16, "UDS RoutineControl Data":u8[], "UDS RoutineControl Read Data":u8[], "Routine Control Mode":u8, "SupportFDCAN":bool, "time config":cluster{"p2_timeout":i32, "p2_extended":i32, "s3_servertime":i32, "s3_clienttime":i32}, "ServiceLayer":cluster{"FilledByte":u8, "STMin":i32, "BlockSize":i32, "FCDelay":i32, "MaxLength":i32}, "Request":u8[], "Respond":u8[]}
  T20 = cluster{"Sender":string, "receiver":string, "message":string, "data":variant}
  T21 = typedef "LVPointTypeDef.ctl" = cluster{"Horizontal":i16, "Vertical":i16}
  T22 = cluster{"MessageName":string, "SignalList":T10[]}[]
  T23 = enum8{"Enabled", "Disabled", "Disabled and Grayed Out"}
  T24 = typedef "TLibCAN.ctl" = cluster{"AIdxchn":u8, "AId":i32, "AIsStd":u8, "AIsData":u8, "ADLC":u8, "ADataArray":cluster{"Data0":u8, "Data1":u8, "Data2":u8, "Data3":u8, "Data4":u8, "Data5":u8, "Data6":u8, "Data7":u8}}
  T25 = typedef "TLibCANFD.ctl" = cluster{"AIdxchn":u8, "AId":i32, "AIsStd":u8, "BRS":enum16{"Close", "Open"}, "AIsData":u8, "ADLC":i32, "AIsFD":enum16{"Classic CAN Message", "FD CAN Message"}, "FDatas":cluster{"Initialize array[0]":u8, "Initialize array[1]":u8, "Initialize array[2]":u8, "Initialize array[3]":u8, "Initialize array[4]":u8, "Initialize array[5]":u8, "Initialize array[6]":u8, "Initialize array[7]":u8, "Initialize array[8]":u8, "Initialize array[9]":u8, "Initialize array[10]":u8, "Initialize array[11]":u8, "Initialize array[12]":u8, "Initialize array[13]":u8, "Initialize array[14]":u8, "Initialize array[15]":u8, "Initialize array[16]":u8, "Initialize array[17]":u8, "Initialize array[18]":u8, "Initialize array[19]":u8, "Initialize array[20]":u8, "Initialize array[21]":u8, "Initialize array[22]":u8, "Initialize array[23]":u8, "Initialize array[24]":u8, "Initialize array[25]":u8, "Initialize array[26]":u8, "Initialize array[27]":u8, "Initialize array[28]":u8, "Initialize array[29]":u8, "Initialize array[30]":u8, "Initialize array[31]":u8, "Initialize array[32]":u8, "Initialize array[33]":u8, "Initialize array[34]":u8, "Initialize array[35]":u8, "Initialize array[36]":u8, "Initialize array[37]":u8, "Initialize array[38]":u8, "Initialize array[39]":u8, "Initialize array[40]":u8, "Initialize array[41]":u8, "Initialize array[42]":u8, "Initialize array[43]":u8, "Initialize array[44]":u8, "Initialize array[45]":u8, "Initialize array[46]":u8, "Initialize array[47]":u8, "Initialize array[48]":u8, "Initialize array[49]":u8, "Initialize array[50]":u8, "Initialize array[51]":u8, "Initialize array[52]":u8, "Initialize array[53]":u8, "Initialize array[54]":u8, "Initialize array[55]":u8, "Initialize array[56]":u8, "Initialize array[57]":u8, "Initialize array[58]":u8, "Initialize array[59]":u8, "Initialize array[60]":u8, "Initialize array[61]":u8, "Initialize array[62]":u8, "Initialize array[63]":u8}}
  T26 = cluster{"FIdxChn":u8, "FProperties":u8, "FDLC":u8, "FFDProperties":u8, "FIdentifier":i32, "FTimeUS":u64, "FData":cluster{"[0]":u8, "[1]":u8, "[2]":u8, "[3]":u8, "[4]":u8, "[5]":u8, "[6]":u8, "[7]":u8, "[8]":u8, "[9]":u8, "[10]":u8, "[11]":u8, "[12]":u8, "[13]":u8, "[14]":u8, "[15]":u8, "[16]":u8, "[17]":u8, "[18]":u8, "[19]":u8, "[20]":u8, "[21]":u8, "[22]":u8, "[23]":u8, "[24]":u8, "[25]":u8, "[26]":u8, "[27]":u8, "[28]":u8, "[29]":u8, "[30]":u8, "[31]":u8, "[32]":u8, "[33]":u8, "[34]":u8, "[35]":u8, "[36]":u8, "[37]":u8, "[38]":u8, "[39]":u8, "[40]":u8, "[41]":u8, "[42]":u8, "[43]":u8, "[44]":u8, "[45]":u8, "[46]":u8, "[47]":u8, "[48]":u8, "[49]":u8, "[50]":u8, "[51]":u8, "[52]":u8, "[53]":u8, "[54]":u8, "[55]":u8, "[56]":u8, "[57]":u8, "[58]":u8, "[59]":u8, "[60]":u8, "[61]":u8, "[62]":u8, "[63]":u8}}
  T27 = cluster{"[0]":u8, "[1]":u8, "[2]":u8, "[3]":u8, "[4]":u8, "[5]":u8, "[6]":u8, "[7]":u8, "[8]":u8, "[9]":u8, "[10]":u8, "[11]":u8, "[12]":u8, "[13]":u8, "[14]":u8, "[15]":u8, "[16]":u8, "[17]":u8, "[18]":u8, "[19]":u8, "[20]":u8, "[21]":u8, "[22]":u8, "[23]":u8, "[24]":u8, "[25]":u8, "[26]":u8, "[27]":u8, "[28]":u8, "[29]":u8, "[30]":u8, "[31]":u8, "[32]":u8, "[33]":u8, "[34]":u8, "[35]":u8, "[36]":u8, "[37]":u8, "[38]":u8, "[39]":u8, "[40]":u8, "[41]":u8, "[42]":u8, "[43]":u8, "[44]":u8, "[45]":u8, "[46]":u8, "[47]":u8, "[48]":u8, "[49]":u8, "[50]":u8, "[51]":u8, "[52]":u8, "[53]":u8, "[54]":u8, "[55]":u8, "[56]":u8, "[57]":u8, "[58]":u8, "[59]":u8, "[60]":u8, "[61]":u8, "[62]":u8, "[63]":u8}
  T28 = cluster{"Data0":u8, "Data1":u8, "Data2":u8, "Data3":u8, "Data4":u8, "Data5":u8, "Data6":u8, "Data7":u8}
  T29 = cluster{"SendData[0]":u8, "SendData[1]":u8, "SendData[2]":u8, "SendData[3]":u8, "SendData[4]":u8, "SendData[5]":u8, "SendData[6]":u8, "SendData[7]":u8}
  T30 = cluster{"SendData[0]":u8, "SendData[1]":u8, "SendData[2]":u8, "SendData[3]":u8, "SendData[4]":u8, "SendData[5]":u8, "SendData[6]":u8, "SendData[7]":u8, "SendData[8]":u8, "SendData[9]":u8, "SendData[10]":u8, "SendData[11]":u8, "SendData[12]":u8, "SendData[13]":u8, "SendData[14]":u8, "SendData[15]":u8, "SendData[16]":u8, "SendData[17]":u8, "SendData[18]":u8, "SendData[19]":u8, "SendData[20]":u8, "SendData[21]":u8, "SendData[22]":u8, "SendData[23]":u8, "SendData[24]":u8, "SendData[25]":u8, "SendData[26]":u8, "SendData[27]":u8, "SendData[28]":u8, "SendData[29]":u8, "SendData[30]":u8, "SendData[31]":u8, "SendData[32]":u8, "SendData[33]":u8, "SendData[34]":u8, "SendData[35]":u8, "SendData[36]":u8, "SendData[37]":u8, "SendData[38]":u8, "SendData[39]":u8, "SendData[40]":u8, "SendData[41]":u8, "SendData[42]":u8, "SendData[43]":u8, "SendData[44]":u8, "SendData[45]":u8, "SendData[46]":u8, "SendData[47]":u8, "SendData[48]":u8, "SendData[49]":u8, "SendData[50]":u8, "SendData[51]":u8, "SendData[52]":u8, "SendData[53]":u8, "SendData[54]":u8, "SendData[55]":u8, "SendData[56]":u8, "SendData[57]":u8, "SendData[58]":u8, "SendData[59]":u8, "SendData[60]":u8, "SendData[61]":u8, "SendData[62]":u8, "SendData[63]":u8}
  T31 = enum32{"invalid app kind", "Development System", "Run Time System", "Student Edition", "Embedded LabVIEW", "Evaluation", "Custom"}
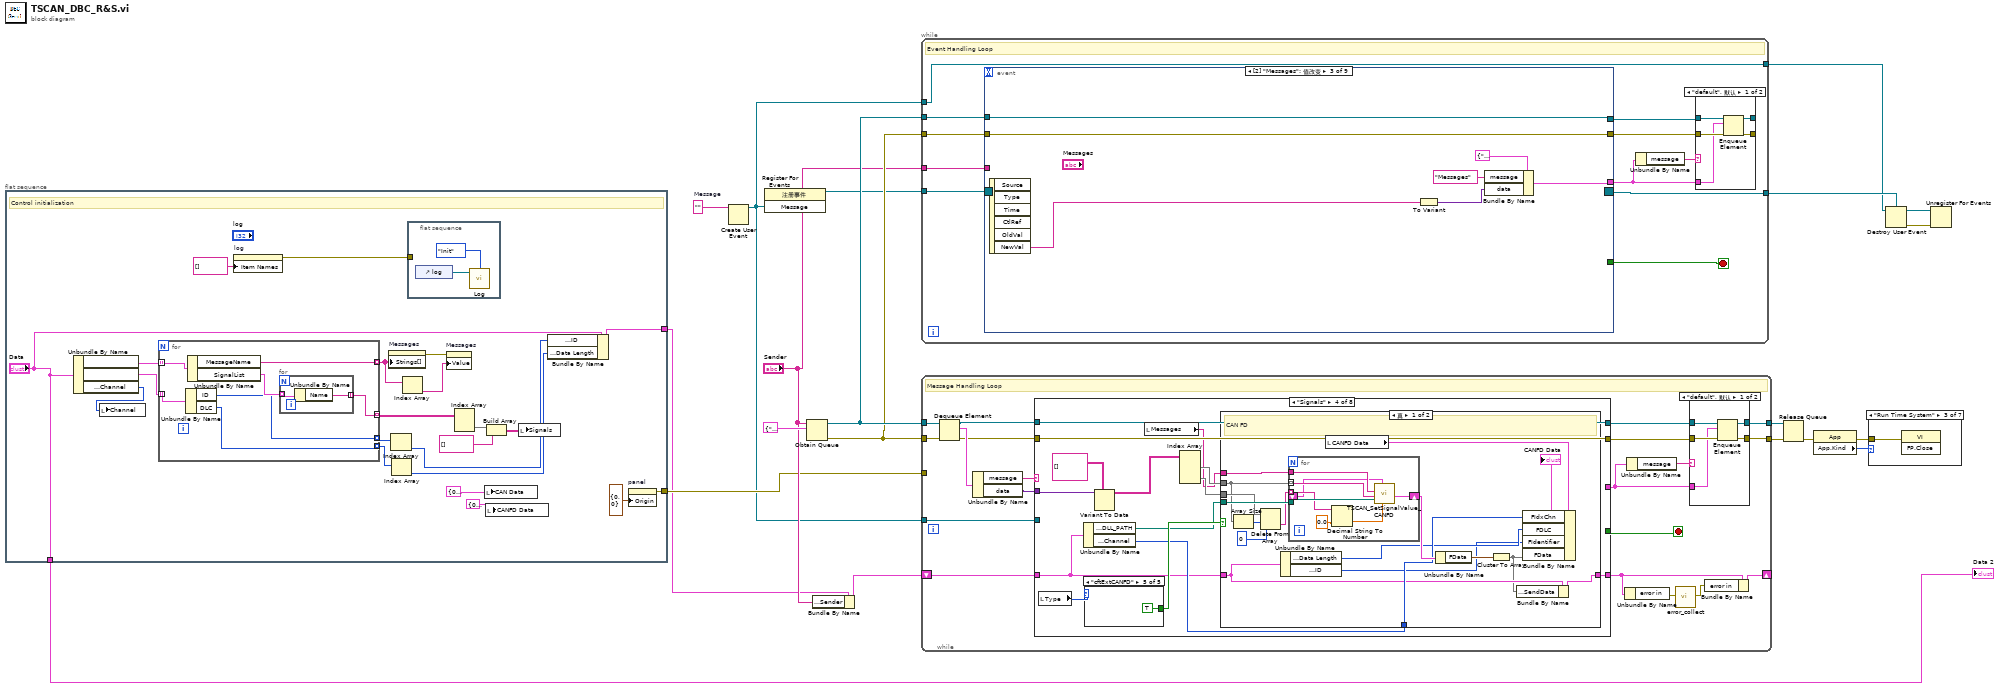
[diagram p0: block diagram]
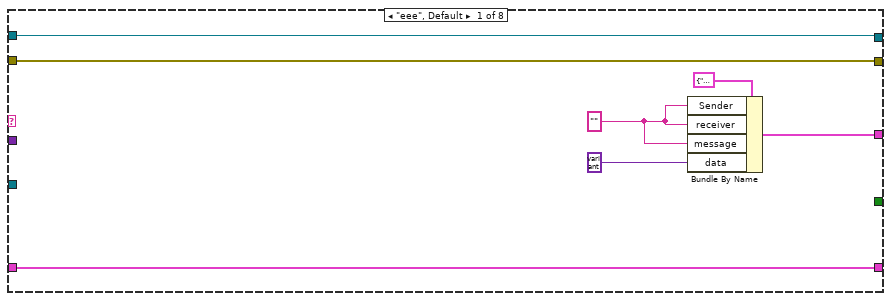
[diagram p9: hidden frame]
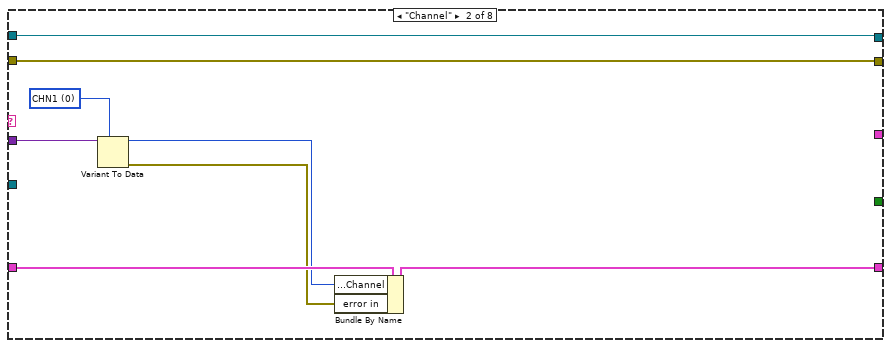
[diagram p10: hidden frame]
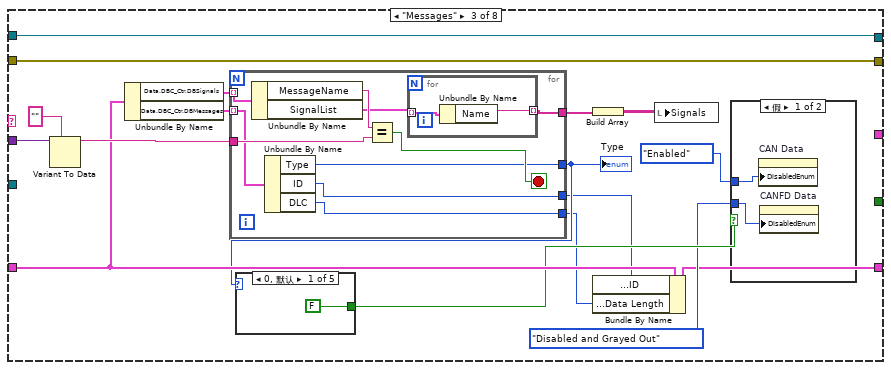
[diagram p11: hidden frame]
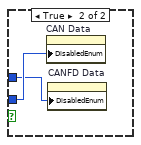
[diagram p12: hidden frame]
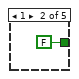
[diagram p13: hidden frame]
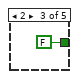
[diagram p14: hidden frame]
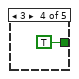
[diagram p15: hidden frame]
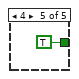
[diagram p16: hidden frame]
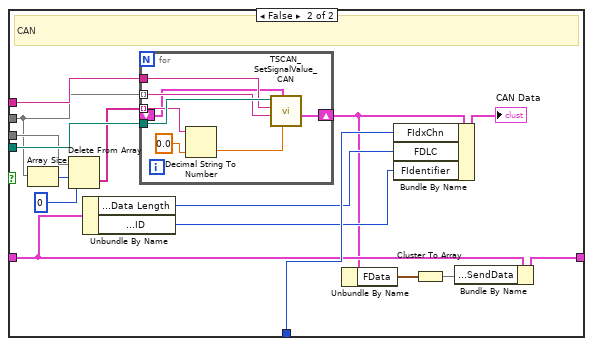
[diagram p17: hidden frame]
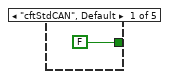
[diagram p18: hidden frame]
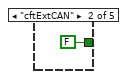
[diagram p19: hidden frame]
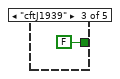
[diagram p20: hidden frame]
diagram:
  w9 = ""  # Message
  n1 = flat-sequence {
    tunnel: [w40] -> w7
    tunnel: [w28] -> w2
    tunnel: ["Data"] -> w1
    frame #0 {
      # "Control initialization"
      n2 = Unbundle By Name("Data") -> ("Data.DBC_Ctr.DBSignals"=w37:T22, "Data.DBC_Ctr.DBMessages"=w27:T9[], "Data.Config_parameter.Channel"=w30:i32)
      n3 = local write "Channel"(w30) -> ()
      n4 = for {
        tunnel: w37 -> [w48] mode=indexing
        tunnel: [w47] -> w35 mode=indexing
        tunnel: [w45] -> w31 mode=indexing
        tunnel: w27 -> [w44] mode=indexing
        tunnel: [w43] -> w26 mode=indexing
        tunnel: [w42] -> w24 mode=indexing
        n5 = Unbundle By Name(w44) -> ("ID"=w43:i32, "DLC"=w42:i32)
        n6 = Unbundle By Name(w48) -> ("MessageName"=w47:string, "SignalList"=w46:T10[])
        n7 = for {
          tunnel: w46 -> [w50] mode=indexing
          tunnel: [w49] -> w45 mode=indexing
          n8 = Unbundle By Name(w50) -> ("Name"=w49:string)
        }
      }
      n9 = property on="log" class="LstBox (严格)"("Item Names"=string[] [] ("项名")) -> (error out=w38:errorcluster)  [unwired: 2 in, 1 out]
      n10 = property on="Messages" class="CmbBox"("Strings[]"=w35) -> (error out=w36:errorcluster)  [unwired: 2 in, 1 out]
      n11 = Index Array(array=w26) -> (element=w25:i32)  [unwired: 1 in]
      n12 = Index Array(array=w24) -> (element=w23:i32)  [unwired: 1 in]
      n13 = Index Array(array=w35) -> (element=w34:string)  [unwired: 1 in]
      n14 = flat-sequence {
        tunnel: w38 -> [_]
        frame #0 {
          n15 = control-ref of="log"() -> (w51:refnum<vi>)
          n16 = call "Log.vi"("Method"=enum16{"Init", "Log"}."Init", "ListBox in"=w51) -> ()  [unwired: 2 in]
        }
      }
      n17 = property on="Messages" class="CmbBox"(error in=w36, "Value"=w34) -> ()  [unwired: 1 in, 2 out]
      n18 = Index Array(array=w31) -> (element=w33:string[])  [unwired: 2 in]
      n19 = local write "CAN Data"(T3 {"FIdxChn"=0, "FProperties"=0, "FDLC"=0, "FReserved"=0, "FIdentifier"=0, "FTimeUS"=0, "FData"={"Data0"=0, "Data1"=0, "Data2"=0, "Data3"=0, "Data4"=0, "Data5"=0, "Data6"=0, "Data7"=0}} ("CAN Data")) -> ()
      n20 = local write "CANFD Data"(T2 {"FIdxChn"=0, "FProperties"=0, "FDLC"=0, "FFDProperties"=0, "FIdentifier"=0, "FTimeUS"=0, "FData"=[]} ("CANFD Data")) -> ()
      n21 = Build Array(w33, string[] [] ("元素")) -> (w32:string[][])
      n22 = local write "Signals"(w32) -> ()
      n23 = Bundle By Name(cluster="Data", "Data.Send_parameter.ID"=w25, "Data.Send_parameter.Data Length"=w23) -> (w28:T4)
      n24 = property on="panel" class="Pane"("Origin"=T21 {"Horizontal"=0, "Vertical"=0} ("原点")) -> (error out=w40:errorcluster)  [unwired: 2 in, 1 out]
    }
  }
  n25 = Create User Event(user event datatype=w9) -> (user event=w4:refnum<user-event>)  [unwired: 1 in, 1 out]
  n26 = register-events(w4) -> (reference out=w8:refnum<event-registration>)  [unwired: 2 in, 1 out]
  n27 = Obtain Queue(name (unnamed)="Sender", element data type=T20 {"Sender"="", "receiver"="", "message"="", "data"=variant} ("Communication message")) -> (queue out=w19:refnum<queue>, error out=w12:errorcluster)  [unwired: 3 in, 1 out]
  n28 = Bundle By Name(cluster=w2, "Communication message.Sender"="Sender") -> (w11:T4)
  n29 = while {
    tunnel: w19 -> [w62]
    tunnel: w12 -> [w60]
    tunnel: "Sender" -> [w56]
    tunnel: w8 -> [w55]
    tunnel: [w54] -> w6
    tunnel: w4 -> [w53]
    tunnel: [w53] -> w3
    stop <- w63 stop-if-true
    # "Event Handling Loop"
    n30 = event shown="[2] \"Messages\": 值改变" {
      selector: w55 -> [_ _ _ _ _ _ _ _ _]
      dyn-events: [_ _ _ _ _ _ _ _ _] -> w54
      timeout: _ -> [_ _ _ _ _ _ _ _ _]
      tunnel: [_ _ _ _ _ _ w106 w111 _] -> w63
      tunnel: w62 -> [w73 w80 w87 w94 w99 w104 w109 w114 w121]
      tunnel: [w73 w80 w87 w94 w99 w104 w109 w112 w121] -> w61
      tunnel: [T20 {"Sender"="", "receiver"="", "message"="", "data"=variant} ("Communication message") w76 w83 w89 w95 w102 _ _ w117] -> w58
      tunnel: [w72 w79 w86 w93 w98 w100 w105 w110 w120] -> w59
      tunnel: w60 -> [w72 w79 w86 w93 w98 w100 w105 w110 w120]
      tunnel: w56 -> [_ _ _ _ _ _ _ _ _]
      event Timeout {
        n31 = event-data() -> ()  [unwired: 1 in, 3 out]
      }
      event "Channel": Value Change {
        n32 = event-data() -> ("NewVal"=w74:i32)  [unwired: 1 in, 5 out]
        n33 = To Variant(anything=w74) -> (Variant=w75:variant)
        n34 = Bundle By Name(cluster=T20 {"Sender"="", "receiver"="", "message"="", "data"=variant} ("Communication message"), "message"="Channel" ("Sender"), "data"=w75) -> (w76:T20)
      }
      event "Messages": Value Change {
        n35 = event-data() -> ("NewVal"=w81:string)  [unwired: 1 in, 5 out]
        n36 = To Variant(anything=w81) -> (Variant=w82:variant)
        n37 = Bundle By Name(cluster=T20 {"Sender"="", "receiver"="", "message"="", "data"=variant} ("Communication message"), "message"="Messages" ("Sender"), "data"=w82) -> (w83:T20)
      }
      event "Signals": Value Change {
        n38 = event-data() -> ("NewVal"=w88:string[][])  [unwired: 1 in, 5 out]
        n39 = To Variant(anything=w88) -> (Variant=w90:variant)
        n40 = Bundle By Name(cluster=T20 {"Sender"="", "receiver"="", "message"="", "data"=variant} ("Communication message"), "message"="Signals" ("Sender"), "data"=w90) -> (w89:T20)
      }
      event "Send": Value Change {
        n41 = event-data() -> ()  [unwired: 1 in, 6 out]
        n42 = Bundle By Name(cluster=T20 {"Sender"="", "receiver"="", "message"="", "data"=variant} ("Communication message"), "message"="Send" ("Sender")) -> (w95:T20)
      }
      event "Quit": Value Change {
        n43 = event-data() -> ()  [unwired: 1 in, 6 out]
        n44 = Bundle By Name(cluster=T20 {"Sender"="", "receiver"="", "message"="", "data"=variant} ("Communication message"), "message"="Quit" ("Sender")) -> (w102:T20)
      }
      event User Event {
        n45 = event-data() -> ("Message"=w108:string)  [unwired: 1 in]
        n46 = Equal?(x=w108, y="Quit") -> (x = y?=w106:bool)
      }
      event Panel Close? {
        w111 = TRUE ("放弃？")
        n47 = event-data() -> ()  [unwired: 1 in, 4 out]
        n48 = Enqueue Element(queue=w114, element=T20 {"Sender"="", "receiver"="", "message"="Quit", "data"=variant} ("Communication message")) -> (queue out=w112:refnum<queue>)  [unwired: 2 in, 2 out]
        n49 = event-data("Discard?"=w111) -> ()  [unwired: 1 in, 1 out]
      }
      event "Creat error": Value Change {
        n50 = event-data() -> ()  [unwired: 1 in, 6 out]
        n51 = To Variant(anything=errorcluster {"status"=TRUE, "code"=709394, "source"="This is a error demo"}) -> (Variant=w115:variant)
        n52 = Bundle By Name(cluster=T20 {"Sender"="", "receiver"="", "message"="", "data"=variant} ("Communication message"), "message"="Creat error" ("Sender"), "data"=w115) -> (w117:T20)
      }
    }
    n53 = Unbundle By Name(w58) -> ("message"=w57:string)
    n54 = case shown="\"default\", 默认" w57 {
      tunnel: w61 -> [w68 w70]
      tunnel: w59 -> [w67 w69]
      tunnel: w58 -> [w66 _]
      tunnel: [w65 w70] -> _
      tunnel: [w64 w69] -> _
      frame "default", Default {
        n55 = Enqueue Element(queue=w68, element=w66, error in (no error)=w67) -> (queue out=w65:refnum<queue>, error out=w64:errorcluster)  [unwired: 1 in, 1 out]
      }
      frame "" {
      }
    }
  }
  n56 = while {
    tunnel: w19 -> [w141]
    tunnel: w12 -> [w140]
    tunnel: [w132] -> w18
    tunnel: [w131] -> w17
    shift-right: [w123] -> _
    shift-left: w11 -> [w127]
    tunnel: w7 -> [_]
    tunnel: w4 -> [w126]
    stop <- w130 stop-if-true
    # "Message Handling Loop"
    n57 = Dequeue Element(queue=w141, error in (no error)=w140) -> (queue out=w137:refnum<queue>, element=w139:T20, error out=w136:errorcluster)  [unwired: 1 in, 1 out]
    n58 = Unbundle By Name(w139) -> ("message"=w138:string, "data"=w133:variant)
    n59 = case shown="\"Signals\"" w138 {
      tunnel: [w155 w163 w180 w215 w275 w327 w334 w341] -> w135
      tunnel: w137 -> [w155 w163 w180 w215 w275 w327 w334 w340]
      tunnel: w136 -> [w154 w162 w179 w214 w274 w326 w333 w338]
      tunnel: [w154 w162 w179 w214 w274 w326 w333 w339] -> w134
      tunnel: w133 -> [_ w160 w178 w213 _ _ w331 _]
      tunnel: [_ _ _ _ _ _ _ TRUE] -> w130
      tunnel: [w152 _ _ _ _ _ _ _] -> w129
      tunnel: [w149 w158 w166 w202 w270 w325 w329 w337] -> w125
      tunnel: w127 -> [w149 w161 w173 w203 w271 w325 w332 w337]
      tunnel: w126 -> [_ _ _ _ _ _ _ w336]
      frame "eee", Default {
        w150 = ""
        n60 = Bundle By Name(cluster=T20 {"Sender"="", "receiver"="", "message"="", "data"=variant} ("Communication message"), "Sender"=w150, "receiver"=w150, "message"=w150, "data"=variant) -> (w152:T20)
      }
      frame "Channel" {
        w159 = 0 items=["CHN1", "CHN2", "CHN3", "CHN4", "CHN5", "CHN6", "CHN7", "CHN8", "CHN9", "CHN10", "CHN11", "CHN12", "CHN13", "CHN14", "CHN15", "CHN16", "CHN17", "CHN18", "CHN19", "CHN20", "CHN21", "CHN22", "CHN23", "CHN24", "CHN25", "CHN26", "CHN27", "CHN28", "CHN29", "CHN30", "CHN31", "CHN32"] ("Channel")
        n61 = Variant To Data(type=w159, Variant=w160) -> (data=w157:i32, error out=w156:errorcluster)  [unwired: 1 in]
        n62 = Bundle By Name(cluster=w161, "Data.Config_parameter.Channel"=w157, "error in"=w156) -> (w158:T4)
      }
      frame "Messages" {
        n63 = Variant To Data(type="", Variant=w178) -> (data=w175:string)  [unwired: 1 in, 1 out]
        n64 = Unbundle By Name(w173) -> ("Data.DBC_Ctr.DBSignals"=w176:T22, "Data.DBC_Ctr.DBMessages"=w174:T9[])
        n65 = for {
          tunnel: w176 -> [w199] mode=indexing
          tunnel: w175 -> [w197]
          tunnel: [w195] -> w172
          tunnel: w174 -> [w194] mode=indexing
          tunnel: [w192] -> w170
          tunnel: [w191] -> w165
          tunnel: [w190] -> w164
          stop <- w193 stop-if-true
          n66 = Unbundle By Name(w199) -> ("MessageName"=w198:string, "SignalList"=w196:T10[])
          n67 = Unbundle By Name(w194) -> ("Type"=w192:u16, "ID"=w191:i32, "DLC"=w190:i32)
          n68 = Equal?(x=w198, y=w197) -> (x = y?=w193:bool)
          n69 = for {
            tunnel: w196 -> [w201] mode=indexing
            tunnel: [w200] -> w195 mode=indexing
            n70 = Unbundle By Name(w201) -> ("Name"=w200:string)
          }
        }
        "Type" <- w170
        n71 = case shown="0, 默认" w170 {
          tunnel: [FALSE FALSE FALSE TRUE TRUE] -> w169
          frame 0, Default {
          }
          frame 1 {
          }
          frame 2 {
          }
          frame 3 {
          }
          frame 4 {
          }
        }
        n72 = Build Array(w172) -> (w171:string[][])
        n73 = Bundle By Name(cluster=w173, "Data.Send_parameter.ID"=w165, "Data.Send_parameter.Data Length"=w164) -> (w166:T4)
        n74 = local write "Signals"(w171) -> ()
        n75 = case shown="假" w169 {
          tunnel: T23."Disabled and Grayed Out" ("禁用") -> [w181 w184]
          tunnel: T23."Enabled" ("禁用") -> [w182 w183]
          frame False {
            n76 = property on="CAN Data" class="Clust (严格)"("DisabledEnum"=w182) -> ()  [unwired: 2 in, 2 out]
            n77 = property on="CANFD Data" class="Clust (严格)"("DisabledEnum"=w181) -> ()  [unwired: 2 in, 2 out]
          }
          frame True {
            n78 = property on="CAN Data" class="Clust (严格)"("DisabledEnum"=w184) -> ()  [unwired: 2 in, 2 out]
            n79 = property on="CANFD Data" class="Clust (严格)"("DisabledEnum"=w183) -> ()  [unwired: 2 in, 2 out]
          }
        }
      }
      frame "Signals" {
        n80 = local read "Type"() -> (w210:T1)
        n81 = Unbundle By Name(w203) -> ("Data.Config_parameter.DLL_PATH"=w208:path, "Data.Config_parameter.Channel"=w204:i32)
        n82 = case shown="\"cftExtCANFD\"" w210 {
          tunnel: [FALSE FALSE FALSE TRUE TRUE] -> w209
          frame "cftStdCAN", Default {
          }
          frame "cftExtCAN" {
          }
          frame "cftJ1939" {
          }
          frame "cftStdCANFD" {
          }
          frame "cftExtCANFD" {
          }
        }
        n83 = Variant To Data(type=string[][] [] ("新值"), Variant=w213) -> (data=w211:string[][])  [unwired: 1 in, 1 out]
        n84 = local read "Messages"() -> (w205:string)
        n85 = Index Array(array=w211) -> (element #1=w207:string[], element #2=w206:string[])  [unwired: 4 in]
        n86 = case shown="真" w209 {
          tunnel: w208 -> [w232 w256]
          tunnel: w207 -> [w229 w253]
          tunnel: w206 -> [w230 w254]
          tunnel: w205 -> [w231 w255]
          tunnel: w204 -> [w221 w248]
          tunnel: w203 -> [w218 w245]
          tunnel: [w217 w244] -> w202
          frame True {
            # "CAN FD"
            n87 = Array Size(array=w229) -> (size(s)=w228:i32)
            n88 = Delete From Array(array=w230, length=w228, index=0 ("索引")) -> (deleted portion=w226:string[])  [unwired: 1 out]
            n89 = Unbundle By Name(w218) -> ("Data.Send_parameter.Data Length"=w220:i32, "Data.Send_parameter.ID"=w219:i32)
            n90 = for {
              tunnel: w232 -> [w240]
              tunnel: w229 -> [w238] mode=indexing
              tunnel: w231 -> [w239]
              tunnel: w226 -> [w237] mode=indexing
              shift-right: [w234] -> w223
              shift-left: _ -> [w233]
              n91 = Decimal String To Number(string=w237, default (0L)=0.0 ("数值")) -> (number=w236:dbl)  [unwired: 1 in, 1 out]
              n92 = call "TSCAN_SetSignalValue_CANFD.vi"("SigValue"=w236, "TLIBCANFD"=w233, "Signal"=w238, "CANFD Message"=w239, "路径输入"=w240) -> ("CANFDObJ"=w234:T26)  [unwired: 3 in, 3 out]
            }
            n93 = local read "CANFD Data"() -> (w224:T2)
            n94 = Unbundle By Name(w223) -> ("FData"=w222:T27)
            n95 = Cluster To Array(cluster=w222) -> (array=w216:u8[])
            n96 = Bundle By Name(cluster=w218, "Data.Send_parameter.SendData"=w216) -> (w217:T4)
            n97 = Bundle By Name(cluster=w224, "FIdxChn"=w221, "FDLC"=w220, "FIdentifier"=w219, "FData"=w216) -> (→"CANFD Data":T2)
          }
          frame False {
            # "CAN"
            n98 = Array Size(array=w253) -> (size(s)=w252:i32)
            n99 = Delete From Array(array=w254, length=w252, index=0 ("索引")) -> (deleted portion=w250:string[])  [unwired: 1 out]
            n100 = Unbundle By Name(w245) -> ("Data.Send_parameter.Data Length"=w247:i32, "Data.Send_parameter.ID"=w246:i32)
            n101 = for {
              tunnel: w256 -> [w264]
              tunnel: w253 -> [w262] mode=indexing
              tunnel: w255 -> [w263]
              tunnel: w250 -> [w261] mode=indexing
              shift-right: [w258] -> w243
              shift-left: _ -> [w257]
              n102 = Decimal String To Number(string=w261, default (0L)=0.0 ("数值")) -> (number=w260:dbl)  [unwired: 1 in, 1 out]
              n103 = call "TSCAN_SetSignalValue_CAN.vi"("SigValue"=w260, "CANObJ IN"=w257, "Signal"=w262, "CAN Message"=w263, "路径输入"=w264) -> ("CANObJ"=w258:T3)  [unwired: 3 in, 3 out]
            }
            n104 = Unbundle By Name(w243) -> ("FData"=w242:T28)
            n105 = Bundle By Name(cluster=w243, "FIdxChn"=w248, "FDLC"=w247, "FIdentifier"=w246) -> (→"CAN Data":T3)
            n106 = Cluster To Array(cluster=w242) -> (array=w241:u8[])
            n107 = Bundle By Name(cluster=w245, "Data.Send_parameter.SendData"=w241) -> (w244:T4)
          }
        }
      }
      frame "Send" {
        n108 = local read "Type"() -> (w273:T1)
        n109 = case shown="\"cftExtCANFD\"" w273 {
          tunnel: [FALSE FALSE FALSE TRUE TRUE] -> w272
          frame "cftStdCAN", Default {
          }
          frame "cftExtCAN" {
          }
          frame "cftJ1939" {
          }
          frame "cftStdCANFD" {
          }
          frame "cftExtCANFD" {
          }
        }
        n110 = case shown="假" w272 {
          tunnel: w271 -> [w296 w319]
          tunnel: [w296 w319] -> w270
          frame False {
            # "CAN"
            n111 = Unbundle By Name(w296) -> ("Data.Config_parameter.DLL_PATH"=w295:path, "Data.Config_parameter.Channel"=w292:i32, "Data.Send_parameter.ID"=w291:i32, "Data.Send_parameter.Frame Format"=w290:u8, "Data.Send_parameter.Frame Type"=w289:u8, "Data.Send_parameter.Data Length"=w288:i32, "Data.Send_parameter.SendData"=w287:u8[])
            n112 = Array To Cluster(array=w287) -> (cluster=w286:T29)
            n113 = Bundle By Name(cluster=T24 {"AIdxchn"=0, "AId"=0, "AIsStd"=0, "AIsData"=0, "ADLC"=0, "ADataArray"={"Data0"=0, "Data1"=0, "Data2"=0, "Data3"=0, "Data4"=0, "Data5"=0, "Data6"=0, "Data7"=0}} ("TCAN"), "AIdxchn"=w292, "AId"=w291, "AIsStd"=w290, "AIsData"=w289, "ADLC"=w288, "ADataArray"=w286) -> (w293:T24)
            n114 = call "tsapp_transmit_can_async.vi"("TCAN"=w293, "Path input"=w295) -> ("error output"=w279:errorcluster, "return"=w277:i32, "Path output"=w278:path)  [unwired: 7 in]
            n115 = Equal To 0?(x=w277) -> (x = 0?=w276:bool)
            n116 = call "tsapp_get_error_description.vi"("error in"=w279, "ACount"=w277, "路径输入"=w278) -> ("ErrDes"=w280:string)  [unwired: 6 in, 2 out]
            n117 = Concatenate Strings("Send CAN Message successful  ") -> (w281:string)
            n118 = Concatenate Strings("Send CAN Message fail ", w280) -> (w283:string)
            n119 = Select(t=w281, s=w276, f=w283) -> (s? t:f=w282:string)
            n120 = call "Log.vi"("Data"=w282) -> ()  [unwired: 3 in]
          }
          frame True {
            # "CANFD"
            n121 = Unbundle By Name(w319) -> ("Data.Config_parameter.DLL_PATH"=w318:path, "Data.Config_parameter.Channel"=w315:i32, "Data.Send_parameter.ID"=w314:i32, "Data.Send_parameter.Frame Format"=w310:u8, "Data.Send_parameter.Frame Type"=w309:u8, "Data.Send_parameter.BRS"=w311:enum16{"Close", "Open"}, "Data.Send_parameter.Data Length"=w307:i32, "Data.Send_parameter.FD Frame"=w308:u8, "Data.Send_parameter.SendData"=w313:u8[])
            n122 = Array To Cluster(array=w313) -> (cluster=w312:T30)
            n123 = Bundle By Name(cluster=T25 {"AIdxchn"=0, "AId"=0, "AIsStd"=0, "BRS"=enum."Close", "AIsData"=0, "ADLC"=0, "AIsFD"=enum."Classic CAN Message", "FDatas"={"Initialize array[0]"=0, "Initialize array[1]"=0, "Initialize array[2]"=0, "Initialize array[3]"=0, "Initialize array[4]"=0, "Initialize array[5]"=0, "Initialize array[6]"=0, "Initialize array[7]"=0, "Initialize array[8]"=0, "Initialize array[9]"=0, "Initialize array[10]"=0, "Initialize array[11]"=0, "Initialize array[12]"=0, "Initialize array[13]"=0, "Initialize array[14]"=0, "Initialize array[15]"=0, "Initialize array[16]"=0, "Initialize array[17]"=0, "Initialize array[18]"=0, "Initialize array[19]"=0, "Initialize array[20]"=0, "Initialize array[21]"=0, "Initialize array[22]"=0, "Initialize array[23]"=0, "Initialize array[24]"=0, "Initialize array[25]"=0, "Initialize array[26]"=0, "Initialize array[27]"=0, "Initialize array[28]"=0, "Initialize array[29]"=0, "Initialize array[30]"=0, "Initialize array[31]"=0, "Initialize array[32]"=0, "Initialize array[33]"=0, "Initialize array[34]"=0, "Initialize array[35]"=0, "Initialize array[36]"=0, "Initialize array[37]"=0, "Initialize array[38]"=0, "Initialize array[39]"=0, "Initialize array[40]"=0, "Initialize array[41]"=0, "Initialize array[42]"=0, "Initialize array[43]"=0, "Initialize array[44]"=0, "Initialize array[45]"=0, "Initialize array[46]"=0, "Initialize array[47]"=0, "Initialize array[48]"=0, "Initialize array[49]"=0, "Initialize array[50]"=0, "Initialize array[51]"=0, "Initialize array[52]"=0, "Initialize array[53]"=0, "Initialize array[54]"=0, "Initialize array[55]"=0, "Initialize array[56]"=0, "Initialize array[57]"=0, "Initialize array[58]"=0, "Initialize array[59]"=0, "Initialize array[60]"=0, "Initialize array[61]"=0, "Initialize array[62]"=0, "Initialize array[63]"=0}} ("TCANFD"), "AIdxchn"=w315, "AId"=w314, "AIsStd"=w310, "BRS"=w311, "AIsData"=w309, "ADLC"=w307, "AIsFD"=w308, "FDatas"=w312) -> (w316:T25)
            n124 = call "tsapp_transmit_canfd_async.vi"("TCANFD"=w316, "Path"=w318) -> ("error out"=w299:errorcluster, "return"=w298:i32, "Path output"=w300:path)  [unwired: 7 in]
            n125 = Equal To 0?(x=w298) -> (x = 0?=w297:bool)
            n126 = call "tsapp_get_error_description.vi"("error in"=w299, "ACount"=w298, "路径输入"=w300) -> ("ErrDes"=w303:string)  [unwired: 6 in, 2 out]
            n127 = Concatenate Strings("Send CANFD Message successful  ") -> (w304:string)
            n128 = Concatenate Strings("Send CANFD Message fail ", w303) -> (w306:string)
            n129 = Select(t=w304, s=w297, f=w306) -> (s? t:f=w305:string)
            n130 = call "Log.vi"("Data"=w305) -> ()  [unwired: 3 in]
          }
        }
      }
      frame "Init" {
      }
      frame "Creat error" {
        n131 = Variant To Data(type=errorcluster {"status"=FALSE, "code"=0, "source"=""} ("error out"), Variant=w331) -> (data=w328:errorcluster)  [unwired: 1 in, 1 out]
        n132 = Bundle By Name(cluster=w332, "error in"=w328) -> (w329:T4)
      }
      frame "Quit" {
        w335 = "Quit" ("y")
        n133 = Generate User Event(user event=w336, event data cluster=w335) -> ()  [unwired: 2 in, 2 out]
        n134 = call "Log.vi"("Data"=w335) -> ()  [unwired: 3 in]
        n135 = Flush Queue(queue=w340, error in (no error)=w338) -> (queue out=w341:refnum<queue>, error out=w339:errorcluster)  [unwired: 1 out]
      }
    }
    n136 = Unbundle By Name(w125) -> ("error in"=w124:errorcluster)
    n137 = Unbundle By Name(w129) -> ("message"=w128:string)
    n138 = call "error_collect.vi"("error in (no error)"=w124) -> ("error IO"=w122:errorcluster)  [unwired: 10 in]
    n139 = case shown="\"default\", 默认" w128 {
      tunnel: w135 -> [w146 w148]
      tunnel: w134 -> [w145 w147]
      tunnel: w129 -> [w144 _]
      tunnel: [w143 w148] -> w132
      tunnel: [w142 w147] -> w131
      frame "default", Default {
        n140 = Enqueue Element(queue=w146, element=w144, error in (no error)=w145) -> (queue out=w143:refnum<queue>, error out=w142:errorcluster)  [unwired: 1 in, 1 out]
      }
      frame "" {
      }
    }
    n141 = Bundle By Name(cluster=w125, "error in"=w122) -> (w123:T4)
  }
  n142 = Release Queue(queue=w18, error in (no error)=w17) -> (error out=w16:errorcluster)  [unwired: 1 in, 2 out]
  n143 = property class="App"(error in=w16) -> (error out=w15:errorcluster, "App.Kind"=w14:T31)  [unwired: 1 in, 1 out]
  n144 = case shown="\"Run Time System\"" w14 {
    tunnel: w15 -> [_ _ w343 _ _ _ _]
    frame "invalid app kind", Default {
    }
    frame "Development System" {
    }
    frame "Run Time System" {
      n145 = invoke class="VI" method="FP.Close"(error in=w343) -> ()  [unwired: 2 in, 3 out]
    }
    frame "Student Edition" {
    }
    frame "Embedded LabVIEW" {
    }
    frame "Evaluation" {
    }
    frame "Custom" {
    }
  }
  n146 = Destroy User Event(user event=w3) -> (error out=w5:errorcluster)  [unwired: 1 in]
  n147 = Unregister For Events(event registration refnum=w6, error in=w5) -> ()  [unwired: 1 out]
  "Data 2" <- w1
